vi "init.vi"(8 "error in (no error)":errorcluster, 11 "DesktopModbus in":refnum<class "DesktopModbus.lvclass">) -> (0 "error out":errorcluster, 3 "DesktopModbus out":refnum<class "DesktopModbus.lvclass">)   [LabVIEW 2015, in "DesktopModbus.lvclass"]
uses:
  DesktopModbus.lvclass
  DesktopModbus.lvclass/DesktopModbus.ctl
  <vilib>/Instr/_visa.llb/VISA Configure Serial Port (Instr).vi
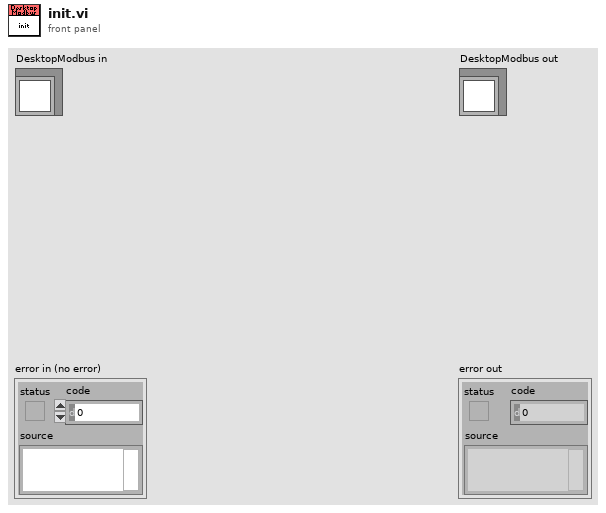
[diagram p1: front panel]
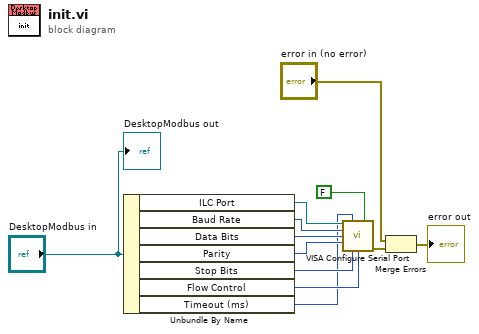
[diagram p0: block diagram]
diagram:
  n1 = Unbundle By Name("DesktopModbus in") -> ("ILC Port"=w7:refnum<visa-resource-name>, "Baud Rate"=w8:u32, "Data Bits"=w9:u16, "Parity"=w10:enum16{"None", "Odd", "Even", "Mark", "Space"}, "Stop Bits"=w11:u16, "Flow Control"=w12:u16, "Timeout (ms)"=w6:u32)
  n2 = call-poly "VISA Configure Serial Port"("VISA resource name"=w7, "timeout (10sec)"=w6, "Enable Termination\nChar (T)"=FALSE ("Enable Termination\nChar (T)"), "baud rate (9600)"=w8, "data bits (8)"=w9, "parity (0:none)"=w10, "stop bits (10: 1 bit)"=w11, "flow control (0:none)"=w12) -> ("error out"=w5:errorcluster)  [unwired: 6 in, 1 out]
  n3 = Merge Errors("error in (no error)", w5) -> (→"error out":errorcluster)
  "DesktopModbus out" <- "DesktopModbus in"
